vi "Parse Command.vi"(11 "command":string) -> (1 "Strings":string[](array[string]), 2 "numbers":dbl[](array[numeric]), 3 "Command":string)   [LabVIEW 2014]
doc: "Used to parse command from producer in the following formats:\n\nCommand (semicolon ;) \nnumbers are seperated by comma (,)\nstrings are seperated by slash( /)\n\nExample:\ncommand;1,2/string/string/"
panel:
  out "first subarray":string[](array[string])
  # "Used to Parse Commands between producer and consumer"
  # "Inputs"
  # "Outputs"
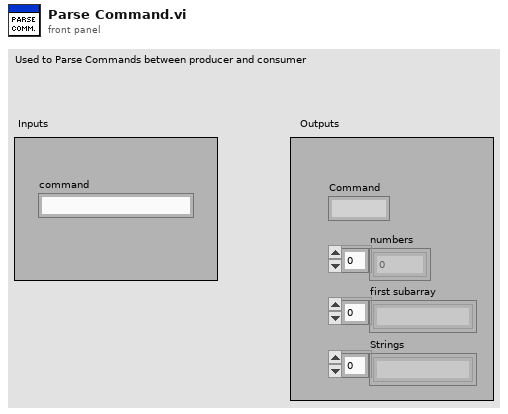
[diagram p1: front panel]
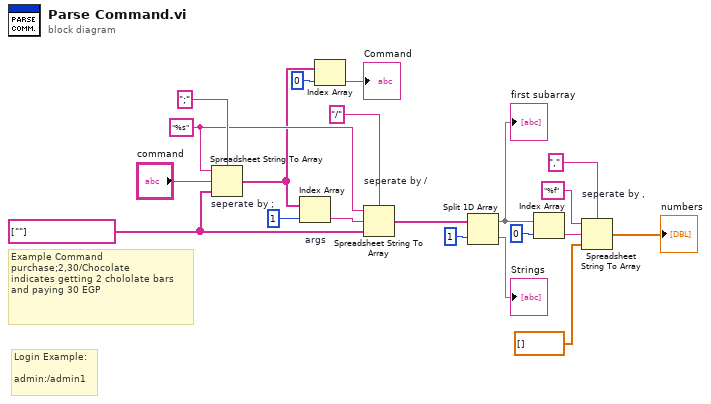
[diagram p0: block diagram]
diagram:
  w13 = string[] [""]
  w17 = "%s" ("format string")
  # "Login Example:\n\nadmin:/admin1"
  # "Example Command\npurchase;2,30/Chocolate\nindicates getting 2 chololate bars and paying 30 EGP"
  n1 = Spreadsheet String To Array "seperate by ;"(delimiter (Tab)=";", format string=w17, spreadsheet string="command", array type (2D Dbl)=w13) -> (array=w3:string[])
  n2 = Index Array "args"(array=w3, index=1) -> (element=w18:string)
  n3 = Index Array(array=w3, index=0) -> (element=→"Command":string)
  n4 = Spreadsheet String To Array "seperate by /"(delimiter (Tab)="/", format string=w17, spreadsheet string=w18, array type (2D Dbl)=w13) -> (array=w12:string[])
  n5 = Split 1D Array(array=w12, index=1) -> (first subarray=w9:string[], second subarray=→"Strings":string[])
  "first subarray" <- w9
  n6 = Index Array(array=w9, index=0) -> (element=w7:string)
  n7 = Spreadsheet String To Array "seperate by ,"(delimiter (Tab)=",", format string="%f", spreadsheet string=w7, array type (2D Dbl)=dbl[] []) -> (array=→"numbers":dbl[])
